vi "Write Command Responses.vi"(8 "error in (no error)":errorcluster, 10 "Command Responses":variant, 11 "Simulado in":refnum<class "Simulado.lvclass">) -> (0 "error out":errorcluster, 3 "Simulado out":refnum<class "Simulado.lvclass">)   [LabVIEW 2020, in "Simulado.lvclass"]
uses:
  Simulado.lvclass
  Simulado.lvclass/Simulado.ctl
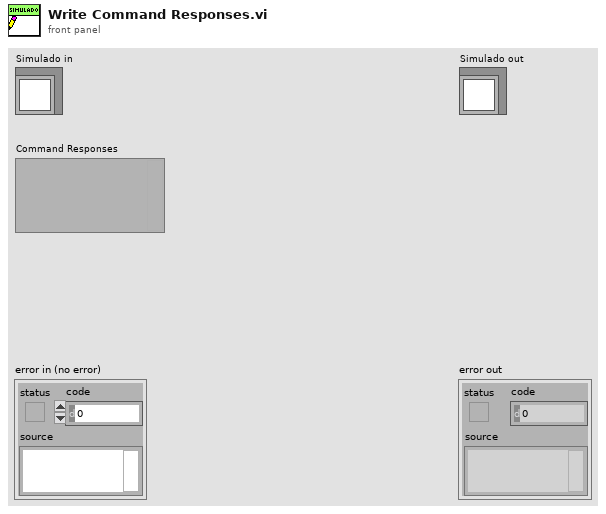
[diagram p1: front panel]
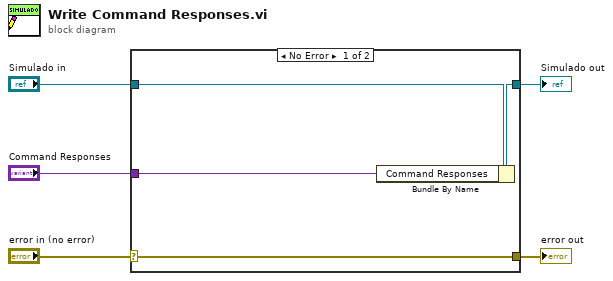
[diagram p0: block diagram]
diagram:
  n1 = case shown="No Error" "error in (no error)" {
    selector: "error in (no error)" -> [w9 w10]
    tunnel: [w9 w10] -> w4
    tunnel: [w7 w11] -> w2
    tunnel: "Simulado in" -> [w8 w11]
    tunnel: "Command Responses" -> [w6 _]
    frame No Error {
      n2 = Bundle By Name(cluster=w8, "Command Responses"=w6) -> (w7:refnum<class "Simulado.lvclass">)
    }
    frame Error {
    }
  }
  "error out" <- w4
  "Simulado out" <- w2
